vi "Read.vi"(6 "RH?":bool, 8 "error in (no error)":errorcluster) -> (0 "error out":errorcluster, 3 "output cluster":T1)   [LabVIEW 2017]
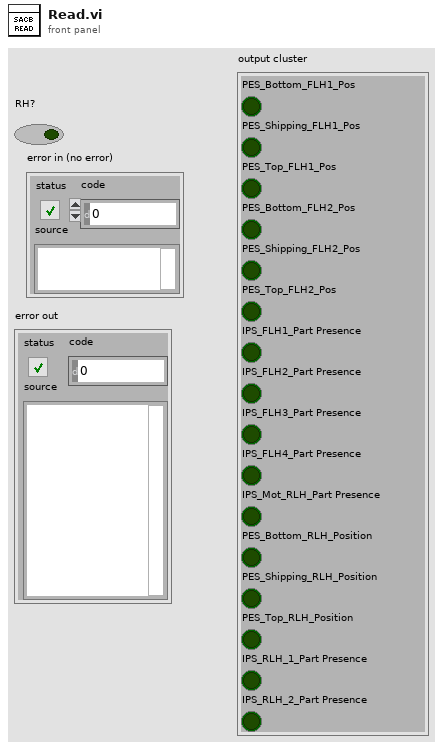
[diagram p1: front panel]
types:
  T1 = cluster{"PES_Bottom_FLH1_Pos":bool, "PES_Shipping_FLH1_Pos":bool, "PES_Top_FLH1_Pos":bool, "PES_Bottom_FLH2_Pos":bool, "PES_Shipping_FLH2_Pos":bool, "PES_Top_FLH2_Pos":bool, "IPS_FLH1_Part Presence":bool, "IPS_FLH2_Part Presence":bool, "IPS_FLH3_Part Presence":bool, "IPS_FLH4_Part Presence":bool, "IPS_Mot_RLH_Part Presence":bool, "PES_Bottom_RLH_Position":bool, "PES_Shipping_RLH_Position":bool, "PES_Top_RLH_Position":bool, "IPS_RLH_1_Part Presence":bool, "IPS_RLH_2_Part Presence":bool}
  T2 = cluster{"C0":bool, "C1":bool, "C2":bool, "C3":bool, "C4":bool, "C5":bool, "C6":bool, "C7":bool, "C8":bool}
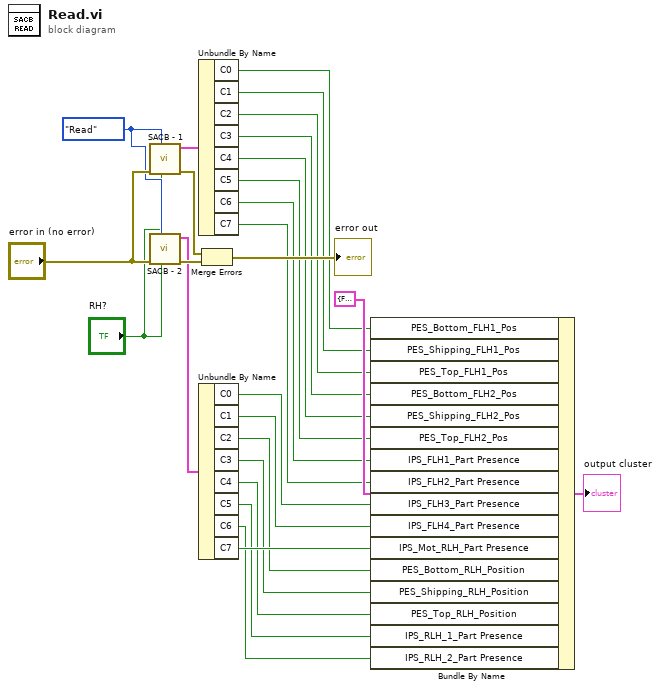
[diagram p0: block diagram]
diagram:
  w25 = enum16{"Create", "Read", "Close"}."Read" ("Command")
  n1 = call "SACB - 1.vi"("RH?"="RH?", "Command"=w25, "Error In"="error in (no error)") -> ("Error Out"=w24:errorcluster, "Digital Inputs"=w22:T2)  [unwired: 7 in]
  n2 = call "SACB - 2.vi"("RH?"="RH?", "Command"=w25, "Error In"="error in (no error)") -> ("Error Out"=w23:errorcluster, "Digital Inputs"=w21:T2)  [unwired: 7 in]
  n3 = Unbundle By Name(w22) -> ("C0"=w2:bool, "C1"=w3:bool, "C2"=w4:bool, "C3"=w5:bool, "C4"=w6:bool, "C5"=w7:bool, "C6"=w8:bool, "C7"=w9:bool)
  n4 = Unbundle By Name(w21) -> ("C0"=w10:bool, "C1"=w11:bool, "C2"=w12:bool, "C3"=w13:bool, "C4"=w14:bool, "C5"=w15:bool, "C6"=w16:bool, "C7"=w17:bool)
  n5 = Merge Errors(w24, w23) -> (→"error out":errorcluster)
  n6 = Bundle By Name(cluster=T1 {"PES_Bottom_FLH1_Pos"=FALSE, "PES_Shipping_FLH1_Pos"=FALSE, "PES_Top_FLH1_Pos"=FALSE, "PES_Bottom_FLH2_Pos"=FALSE, "PES_Shipping_FLH2_Pos"=FALSE, "PES_Top_FLH2_Pos"=FALSE, "IPS_FLH1_Part Presence"=FALSE, "IPS_FLH2_Part Presence"=FALSE, "IPS_FLH3_Part Presence"=FALSE, "IPS_FLH4_Part Presence"=FALSE, "IPS_Mot_RLH_Part Presence"=FALSE, "PES_Bottom_RLH_Position"=FALSE, "PES_Shipping_RLH_Position"=FALSE, "PES_Top_RLH_Position"=FALSE, "IPS_RLH_1_Part Presence"=FALSE, "IPS_RLH_2_Part Presence"=FALSE} ("output cluster"), "PES_Bottom_FLH1_Pos"=w2, "PES_Shipping_FLH1_Pos"=w3, "PES_Top_FLH1_Pos"=w4, "PES_Bottom_FLH2_Pos"=w5, "PES_Shipping_FLH2_Pos"=w6, "PES_Top_FLH2_Pos"=w7, "IPS_FLH1_Part Presence"=w8, "IPS_FLH2_Part Presence"=w9, "IPS_FLH3_Part Presence"=w10, "IPS_FLH4_Part Presence"=w11, "IPS_Mot_RLH_Part Presence"=w17, "PES_Bottom_RLH_Position"=w12, "PES_Shipping_RLH_Position"=w13, "PES_Top_RLH_Position"=w14, "IPS_RLH_1_Part Presence"=w15, "IPS_RLH_2_Part Presence"=w16) -> (→"output cluster":T1)
